vi "Actor Core.vi"(8 "error in":errorcluster, 11 "Actor_UI_Template in":refnum<class "Actor_UI_Template.lvclass">) -> (0 "error out":errorcluster, 3 "Actor out":refnum<class "Actor.lvclass">)   [LabVIEW 2020, in "Actor_UI_Template.lvlib" / "Actor_UI_Template.lvclass"]
doc: "(<B>Filename</B>: Actor Framework.lvlib:Actor.lvclass:Actor Core.vi)\n\nReceives messages to the actor, reacts to them, and initiates any error handling that may shut the actor down.\n\nDescendant classes may override this VI to append parallel tasks for the actor to complete while it handles messages. Overrides use the Call Parent Class Method node."
uses:
  Actor_UI_Template.lvclass
  C:/Program Files/National Instruments/LabVIEW 2020/vi.lib/ActorFramework/Actor/Actor.lvclass
  <vilib>/ActorFramework/Actor/Actor.lvclass
  Actor_UI_Template.lvclass/Actor_UI_Template.ctl
  UI Event Enum.ctl
  <vilib>/ActorFramework/Actor/Actor.lvclass/Actor.ctl
  I_UI_Events Messages/UI Events On Msg/UI Events On Msg.lvclass/UI Events On Msg.ctl
  <vilib>/ActorFramework/Message Enqueuer/Message Enqueuer.lvclass/Message Enqueuer.ctl
  <vilib>/ActorFramework/Stop Msg/Stop Msg.lvclass/Stop Msg.ctl
  <vilib>/ActorFramework/Message Enqueuer/Enqueue.vi
  <vilib>/ActorFramework/Message Enqueuer/Init from Existing Queue.vi
  <vilib>/ActorFramework/Stop Msg/Send Emergency Stop.vi
  <vilib>/ActorFramework/Stop Msg/Send Normal Stop.vi
  <vilib>/ActorFramework/Message Enqueuer/Enqueue Critical.vi
  I_UI_Events Messages/UI Events On Msg/UI Events On Msg.lvclass
  C:/Program Files/National Instruments/LabVIEW 2020/vi.lib/ActorFramework/Message/Message.lvclass
  <vilib>/ActorFramework/Stop Msg/Stop Msg.lvclass
  <vilib>/ActorFramework/Message Priority Queue/Priority Enqueue.vi
  <vilib>/ActorFramework/Message Enqueuer/Message Enqueuer.lvclass
  Actor_UI_Template.lvlib
panel:
  # "This is UI Template, close the panel to exit"
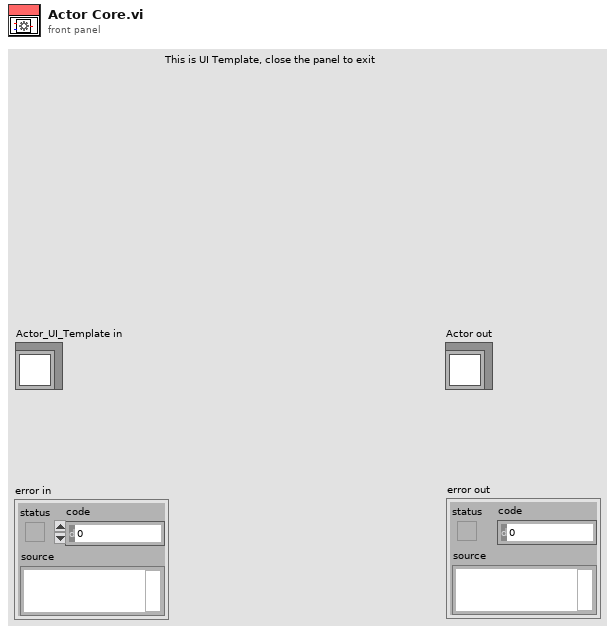
[diagram p1: front panel]
types:
  T1 = enum32{"Invalid", "Standard", "Closed", "Hidden", "Minimized", "Maximized"}
  T2 = typedef "Actor_UI_Template.lvlib/UI Event Enum.ctl" = enum16{"UI Close"}
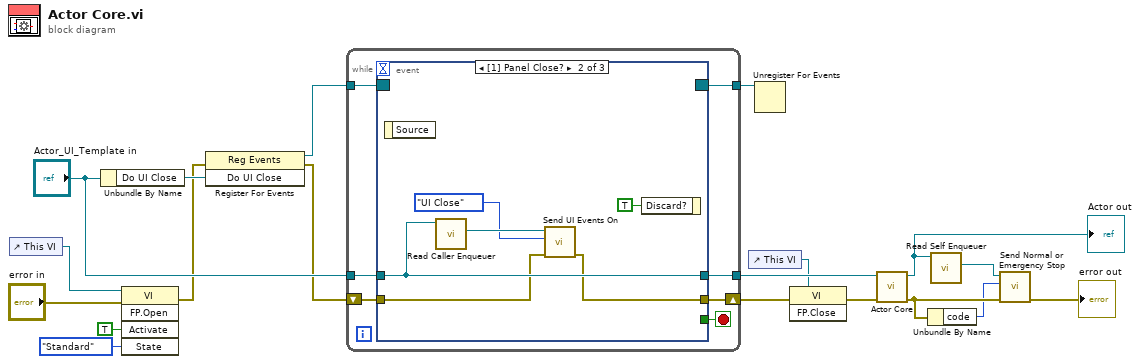
[diagram p0: block diagram]
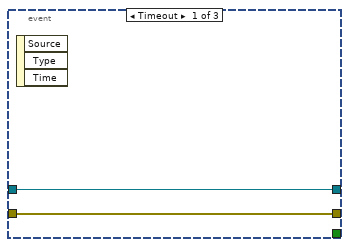
[diagram p2: hidden frame]
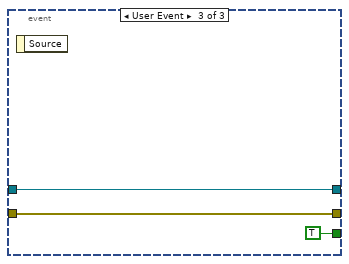
[diagram p3: hidden frame]
diagram:
  n1 = control-ref of="This VI"() -> (w15:refnum<vi>)
  n2 = Unbundle By Name("Actor_UI_Template in") -> ("Do UI Close"=w11:refnum<user-event>)
  n3 = invoke class="VI" method="FP.Open"(reference=w15, error in="error in", "Activate"=TRUE ("Activate?"), "State"=T1."Standard") -> (error out=w10:errorcluster)  [unwired: 1 in, 4 out]
  n4 = register-events(error in=w10, w11) -> (reference out=w16:refnum<event-registration>, error out=w17:errorcluster)  [unwired: 1 in]
  n5 = while {
    tunnel: [w26] -> w19
    tunnel: "Actor_UI_Template in" -> [w25]
    tunnel: w16 -> [w22]
    shift-right: [w24] -> w7
    shift-left: w17 -> [w23]
    tunnel: [w20] -> w1
    stop <- w21 stop-if-true
    n6 = event shown="[1] Panel Close?" {
      selector: w22 -> [_ _ _]
      dyn-events: [_ _ _] -> w20
      timeout: _ -> [_ _ _]
      tunnel: [w28 w33 w37] -> w26
      tunnel: w25 -> [w28 w33 w37]
      tunnel: [w27 w29 w35] -> w24
      tunnel: w23 -> [w27 w30 w35]
      tunnel: [_ _ TRUE] -> w21
      event Timeout {
        n7 = event-data() -> ()  [unwired: 1 in, 3 out]
      }
      event Panel Close? {
        n8 = event-data() -> ()  [unwired: 1 in, 1 out]
        n9 = call <vilib>:"Read Caller Enqueuer.vi"("Actor"=w33) -> ("Caller Enqueuer"=w32:refnum<class "Message Enqueuer.lvclass">)  [unwired: 10 in]
        n10 = call "Send UI Events On.vi"("error in (no error)"=w30, "UI Events"=UI_Event_Enum."UI Close", "Message Enqueuer"=w32) -> ("error out"=w29:errorcluster)  [unwired: 7 in, 1 out]
        n11 = event-data("Discard?"=TRUE) -> ()  [unwired: 1 in, 1 out]
      }
      event User Event {
        n12 = event-data() -> ()  [unwired: 1 in, 1 out]
      }
    }
  }
  n13 = control-ref of="This VI"() -> (w9:refnum<vi>)
  n14 = Unregister For Events(event registration refnum=w1) -> ()  [unwired: 1 in, 1 out]
  n15 = invoke class="VI" method="FP.Close"(reference=w9, error in=w7) -> (error out=w8:errorcluster)  [unwired: 1 in, 2 out]
  n16 = call-parent "Actor Core.vi"("error in"=w8, "Actor in"=w19) -> ("error out"=w3:errorcluster, "Actor out"=w6:refnum<class "Actor.lvclass">)  [unwired: 8 in]
  "Actor out" <- w6
  n17 = Unbundle By Name(w3) -> ("code"=w2:i32)
  n18 = call <vilib>:"Read Self Enqueuer.vi"("Actor"=w6) -> ("Self Enqueuer"=w4:refnum<class "Message Enqueuer.lvclass">)  [unwired: 10 in]
  n19 = call <vilib>:"Send Normal or Emergency Stop.vi"("error in (no error)"=w3, "final error code"=w2, "Message Enqueuer"=w4) -> ("error out"=→"error out":errorcluster)  [unwired: 8 in]
